vi "SetEntryWaveform.vi"(1 "Waveform Name":string, 3 "error in (no error)":errorcluster, 4 "Element":i16=1 min=1, 5 "Channel":u16(ring) items=["Channel 1", "Channel 2", "Channel 3", "Channel 4", "Channel 5", "Channel 6", "Channel 7", "Channel 8", "Digital"], 6 "VISA resource name":refnum<visa-resource-name>) -> (0 "error out":errorcluster, 2 "VISA resource name out":refnum<visa-resource-name>)   [LabVIEW 2020, in "Active Technologies AWG3000.lvlib"]
uses:
  Active Technologies AWG3000.lvlib
panel:
  # "Inserts the waveform present in the Waveform List into the sequencer n-element"
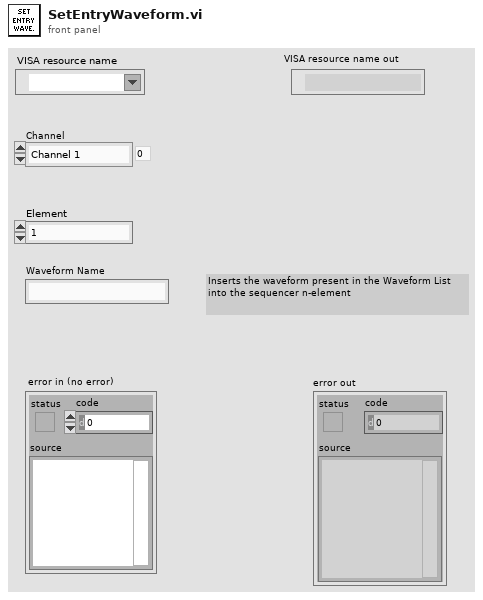
[diagram p1: front panel]
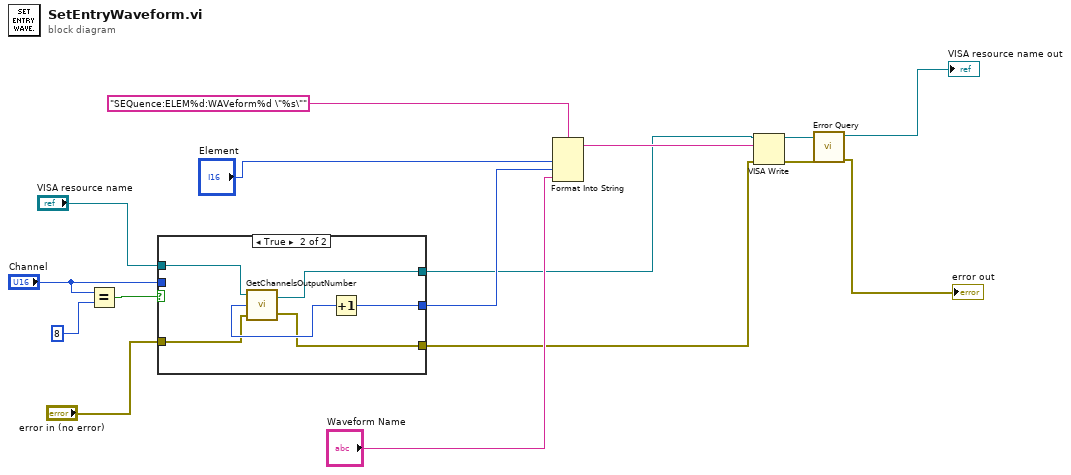
[diagram p0: block diagram]
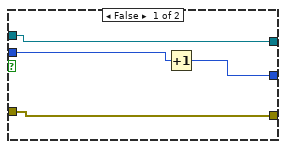
[diagram p2: hidden frame]
diagram:
  n1 = Equal?(x="Channel", y=u16 8) -> (x = y?=w7:bool)
  n2 = case shown="True" w7 {
    tunnel: [w19 w25] -> w6
    tunnel: "error in (no error)" -> [w17 w24]
    tunnel: "VISA resource name" -> [w18 w23]
    tunnel: [w17 w22] -> w3
    tunnel: [w18 w21] -> w2
    tunnel: "Channel" -> [w20 _]
    frame False {
      n3 = Increment(x=w20) -> (x+1=w19:u16)
    }
    frame True {
      n4 = call "GetChannelsOutputNumber.vi"("error in (no error)"=w24, "VISA resource name"=w23) -> ("error out"=w22:errorcluster, "VISA resource name out"=w21:refnum<visa-resource-name>, "Output Channels Number"=w26:i8)
      n5 = Increment(x=w26) -> (x+1=w25:i8)
    }
  }
  n6 = Format Into String(format string="SEQuence:ELEM%d:WAVeform%d \"%s\"" ("write buffer"), "Element", w6, "Waveform Name") -> (resulting string=w9:string)  [unwired: 2 in, 1 out]
  n7 = VISA Write(VISA resource name=w2, write buffer=w9, error in (no error)=w3) -> (VISA resource name out=w15:refnum<visa-resource-name>, error out=w14:errorcluster)  [unwired: 1 out]
  n8 = call "Error Query.vi"("error in (no error)"=w14, "VISA resource name"=w15) -> ("error out"=→"error out":errorcluster, "VISA resource name out"=→"VISA resource name out":refnum<visa-resource-name>)  [unwired: 6 in, 2 out]
